vi "ReportClearLoopError.vi"(7 "reporting process name":string, 8 "error in":errorcluster, 10 "override classification":string, 11 "error reporter":refnum<class "ErrorReporter.lvclass">) -> (0 "cleared error out":errorcluster, 2 "error reported?":bool)   [LabVIEW 2014, in "CLM_ErrorHandler.lvlib" / "ErrorReporter.lvclass"]
uses:
  ErrorReporter.lvclass
  ErrorReporter.lvclass/ErrorReporter.ctl
  ErrorMessage.ctl
  <vilib>/CLM/LocalMessenger/PriorityLocalMessage/CLM_PriorityLocalMessage.lvclass/CLM_PriorityLocalMessage.ctl
  <vilib>/CLM/LocalMessenger/LocalMessage_Queue/CLM_LocalMessage_Queue.lvclass/CLM_LocalMessage_Queue.ctl
  <vilib>/CLM/LocalMessenger/PriorityLocalMessage/SendMessage.vi
  <vilib>/CLM/LocalMessenger/PriorityLocalMessage/SendMessageCluster.vi
  <vilib>/CLM/LocalMessenger/LocalMessage/BundleMessageCluster.vi
  <vilib>/CLM/LocalMessenger/LocalMessage_Queue/SendQueueMessage_Cluster.vi
  <vilib>/CLM/LocalMessenger/PriorityLocalMessage/BufferIndexToPriority.vi
  <vilib>/CLM/LocalMessenger/PriorityLocalMessage/PriorityToBufferIndex.vi
  <vilib>/CLM/LocalMessenger/PriorityLocalMessage/CheckValidReference.vi
  <vilib>/CLM/LocalMessenger/PriorityLocalMessage/CLM_PriorityLocalMessage.lvclass
  CLM_ErrorHandler.lvlib
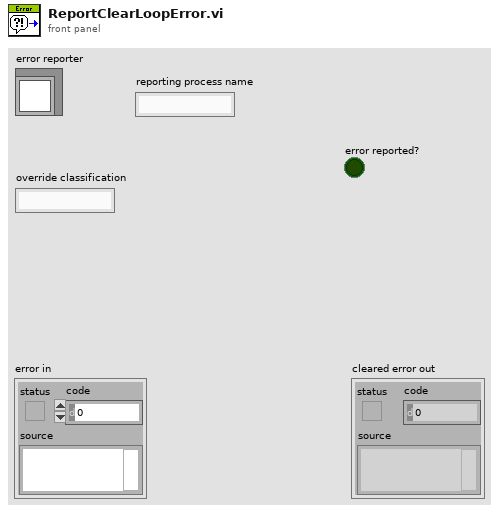
[diagram p1: front panel]
types:
  T1 = typedef "CLM_ErrorHandler.lvlib/ErrorMessage.ctl" = cluster{"error":errorcluster, "classification":string, "time reported":timestamp, "reporting process":string}
  T2 = typedef "CLM_ErrorHandler.lvlib/ErrorReporter.lvclass/ReportingParameter.ctl" = cluster{"error code":i32, "reporting priority":i32, "min dup period (s)":dbl, "classification":string}
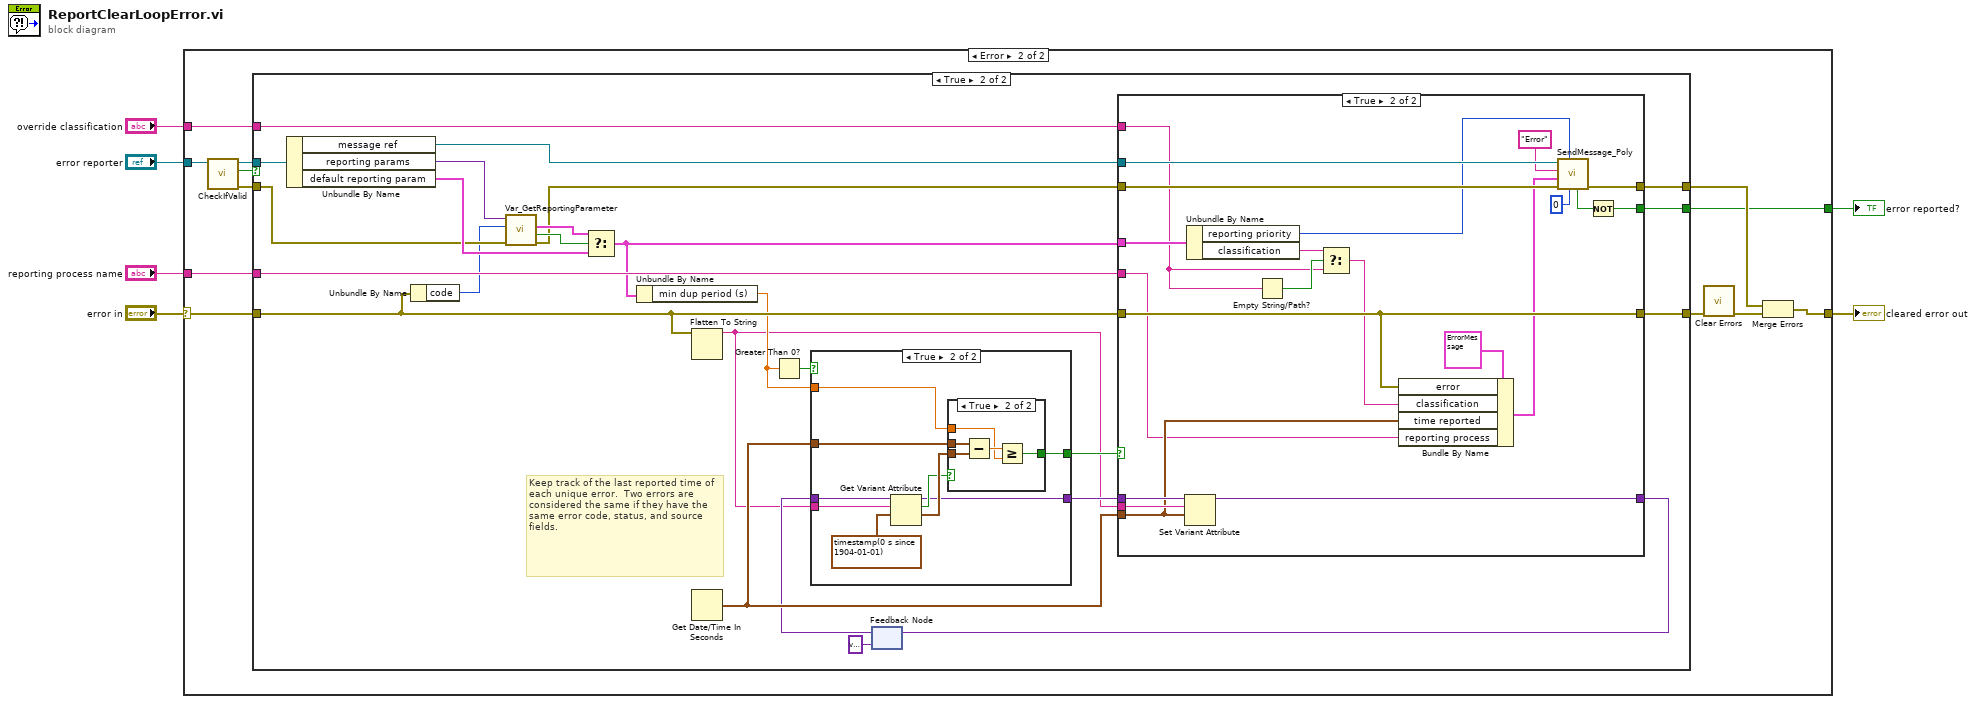
[diagram p0: block diagram]
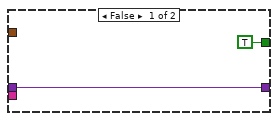
[diagram p5: hidden frame]
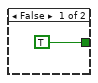
[diagram p6: hidden frame]
diagram:
  n1 = case shown="Error" "error in" {
    selector: "error in" -> [w7 w13]
    tunnel: [w7 w16] -> w5
    tunnel: "error reporter" -> [_ w11]
    tunnel: [_ w15] -> w3
    tunnel: "reporting process name" -> [_ w14]
    tunnel: "override classification" -> [_ w12]
    frame No Error {
    }
    frame Error {
      n2 = call "CheckIfValid.vi"("error reporter in"=w11) -> ("error out"=w8:errorcluster, "valid?"=w9:bool, "error reporter out"=w10:refnum<class "ErrorReporter.lvclass">)  [unwired: 8 in]
      n3 = case shown="True" w9 {
        tunnel: [w21 w44] -> w19
        tunnel: [w20 w43] -> w18
        tunnel: [_ w42] -> w15
        tunnel: w14 -> [_ w41]
        tunnel: w13 -> [w21 w39]
        tunnel: w12 -> [_ w37]
        tunnel: w10 -> [_ w36]
        tunnel: w8 -> [w20 w35]
        frame False {
        }
        frame True {
          # "Keep track of the last reported time of each unique error.  Two errors are considered the same if they have the same error code, status, and source fields."
          n4 = Unbundle By Name(w36) -> ("message ref"=w38:refnum<class "CLM_PriorityLocalMessage.lvclass">, "reporting params"=w46:variant, "default reporting param"=w45:T2)
          n5 = Unbundle By Name(w39) -> ("code"=w22:i32)
          n6 = call "Var_GetReportingParameter.vi"("error in"=w35, "error code"=w22, "reporting params in"=w46) -> ("error out"=w24:errorcluster, "found?"=w34:bool, "reporting parameter"=w33:T2)  [unwired: 5 in, 1 out]
          n7 = Select(t=w33, s=w34, f=w45) -> (s? t:f=w23:T2)
          n8 = Unbundle By Name(w23) -> ("min dup period (s)"=w31:dbl)
          n9 = Flatten To String(anything=w39) -> (data string=w25:string)  [unwired: 3 in, 2 out]
          n10 = Get Date/Time In Seconds() -> (seconds since 1Jan1904=w40:timestamp)
          n11 = Greater Than 0?(x=w31) -> (x > 0?=w32:bool)
          n12 = feedback #1(variant) -> (w30:variant)
          n13 = case shown="True" w32 {
            tunnel: w31 -> [_ w77]
            tunnel: [w72 w75] -> w27
            tunnel: w30 -> [w72 w80]
            tunnel: w40 -> [_ w79]
            tunnel: [TRUE w74] -> w28
            tunnel: w25 -> [_ w73]
            frame False {
            }
            frame True {
              n14 = Get Variant Attribute(Variant=w80, name=w73, default value (empty Variant)=timestamp(0 s since 1904-01-01) ("current time")) -> (duplicate Variant=w75:variant, found=w76:bool, value=w78:timestamp)  [unwired: 1 in, 1 out]
              n15 = case shown="True" w76 {
                tunnel: w79 -> [_ w87]
                tunnel: w78 -> [_ w86]
                tunnel: w77 -> [_ w84]
                tunnel: [TRUE w83] -> w74
                frame False {
                }
                frame True {
                  n16 = Subtract(x=w87, y=w86) -> (x-y=w85:dbl)
                  n17 = Greater Or Equal?(x=w85, y=w84) -> (x >= y?=w83:bool)
                }
              }
            }
          }
          n18 = case shown="True" w28 {
            tunnel: w27 -> [w49 w70]
            tunnel: [w49 w68] -> w26
            tunnel: w25 -> [_ w69]
            tunnel: w40 -> [_ w60]
            tunnel: w39 -> [w47 w63]
            tunnel: w38 -> [_ w67]
            tunnel: w24 -> [w48 w66]
            tunnel: [w48 w65] -> w43
            tunnel: [w47 w63] -> w44
            tunnel: [_ w57] -> w42
            tunnel: w23 -> [_ w62]
            tunnel: w41 -> [_ w58]
            tunnel: w37 -> [_ w50]
            frame False {
            }
            frame True {
              n19 = Set Variant Attribute(Variant=w70, name=w69, value=w60) -> (Variant out=w68:variant)  [unwired: 1 in, 2 out]
              n20 = Unbundle By Name(w62) -> ("reporting priority"=w61:i32, "classification"=w52:string)
              n21 = Empty String/Path?(string/path=w50) -> (empty?=w53:bool)
              n22 = Select(t=w52, s=w53, f=w50) -> (s? t:f=w51:string)
              n23 = Bundle By Name(cluster=T1 {"error"={"status"=FALSE, "code"=0, "source"=""}, "classification"="", "time reported"=timestamp(0 s since 1904-01-01), "reporting process"=""} ("error message"), "error"=w63, "classification"=w51, "time reported"=w60, "reporting process"=w58) -> (w59:T1)
              n24 = call-poly <vilib>:"SendMessage_Poly.vi"("timeout in ms (-1)"=0, "priority (-1, highest)"=w61, "error in"=w66, "data"=w59, "name"="Error", "message ref in"=w67) -> ("error out"=w65:errorcluster, "timed out?"=w54:bool)  [unwired: 2 in, 2 out]
              n25 = Not(x=w54) -> (.not. x?=w57:bool)
            }
          }
          n26 = feedback-in #1(w26) -> ()
        }
      }
      n27 = call <vilib>:"Clear Errors.vi"("error in (no error)"=w19) -> ("error out"=w17:errorcluster)  [unwired: 5 in, 1 out]
      n28 = Merge Errors(w18, w17) -> (w16:errorcluster)
    }
  }
  "cleared error out" <- w5
  "error reported?" <- w3
